vi "Configure Event Search (Serial Bus - UART).vi"(7 "Data Value (0)":i32, 8 "error in (no error)":errorcluster, 9 "Qualifier (0: Equal)":i32(ring) items=["Equal", "Not Equal", "Greater Than", "Less Than"], 10 "Search Operation (0: Rx Data)":i32(ring) items=["Rx Data", "Rx Data 1", "Rx Data 0", "Rx Data X", "Tx Data", "Tx Data 1", "Tx Data 0", "Tx Data X", "Parity Error", "Any Error"], 11 "VISA resource name":refnum<visa-resource-name>) -> (0 "error out":errorcluster, 3 "VISA resource name out":refnum<visa-resource-name>)   [LabVIEW 2017, in "Agilent 2000 3000 X-Series.lvlib"]
doc: "Configures the event search of UART bus.\n\nNotes:\nThis VI is not supported by EDUX1052A/G, DSOX1202A/G, DSOX1204A/G models."
uses:
  Agilent 2000 3000 X-Series.lvlib
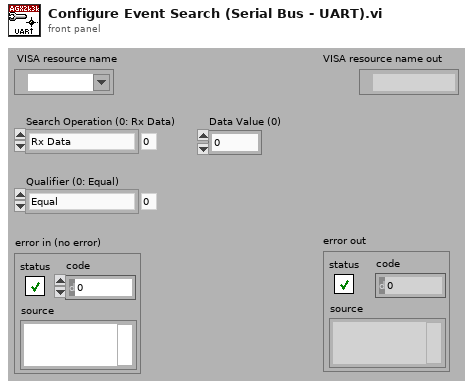
[diagram p1: front panel]
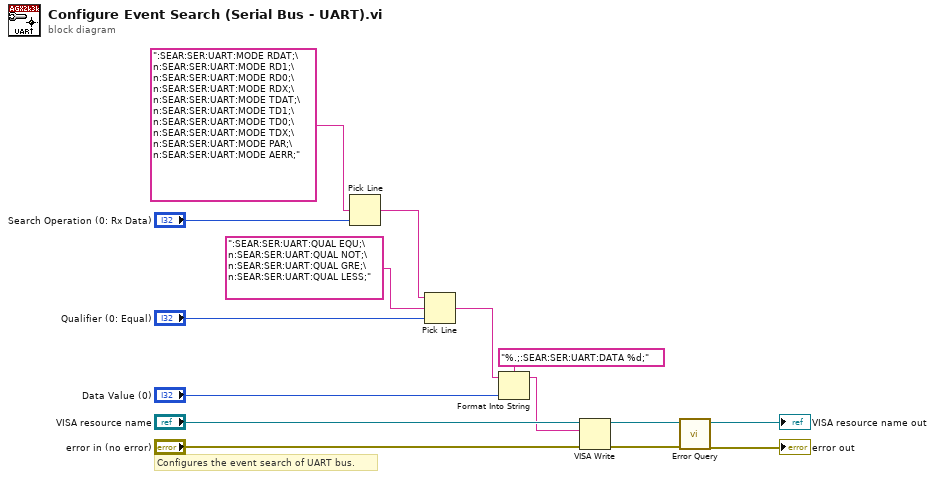
[diagram p0: block diagram]
diagram:
  # "Configures the event search of UART bus."
  n1 = Pick Line(multi-line string=":SEAR:SER:UART:MODE RDAT;\n:SEAR:SER:UART:MODE RD1;\n:SEAR:SER:UART:MODE RD0;\n:SEAR:SER:UART:MODE RDX;\n:SEAR:SER:UART:MODE TDAT;\n:SEAR:SER:UART:MODE TD1;\n:SEAR:SER:UART:MODE TD0;\n:SEAR:SER:UART:MODE TDX;\n:SEAR:SER:UART:MODE PAR;\n:SEAR:SER:UART:MODE AERR;", line index="Search Operation (0: Rx Data)") -> (output string=w9:string)  [unwired: 1 out]
  n2 = Pick Line(string ("")=w9, multi-line string=":SEAR:SER:UART:QUAL EQU;\n:SEAR:SER:UART:QUAL NOT;\n:SEAR:SER:UART:QUAL GRE;\n:SEAR:SER:UART:QUAL LESS;", line index="Qualifier (0: Equal)") -> (output string=w2:string)
  n3 = Format Into String(format string="%.;:SEAR:SER:UART:DATA %d;", initial string=w2, "Data Value (0)") -> (resulting string=w1:string)  [unwired: 1 in, 1 out]
  n4 = VISA Write(VISA resource name="VISA resource name", write buffer=w1, error in (no error)="error in (no error)") -> (VISA resource name out=w6:refnum<visa-resource-name>, error out=w5:errorcluster)  [unwired: 1 out]
  n5 = call "Error Query.vi"("error in (no error)"=w5, "VISA resource name"=w6) -> ("error out"=→"error out":errorcluster, "VISA resource name out"=→"VISA resource name out":refnum<visa-resource-name>)  [unwired: 8 out]
